vi "Simple Spectrometer Demo.vi"() -> ()   [LabVIEW 2010]
uses:
  C:/Users/User/Desktop/LabView/RgbDriverKit.dll
  RgbDriverKit.dll
panel:
  out "Device":string
  out "Measured spectrum":cluster{"Y":dbl[], "Y":dbl[]}[](graph)
  out "error out":errorcluster
  in  "error in (no error)":errorcluster
  out "Status":i32(ring) items=["Idle"=0, "WaitingForTrigger"=1, "TakingSpectrum"=2, "HasData"=3, "Error"=-3, "Busy"=-2, "NotReady"=-1]
  in  "Use sensitivity calibration":bool
  in  "Exposure time [sec]":dbl=0.1 format="%#_6f"
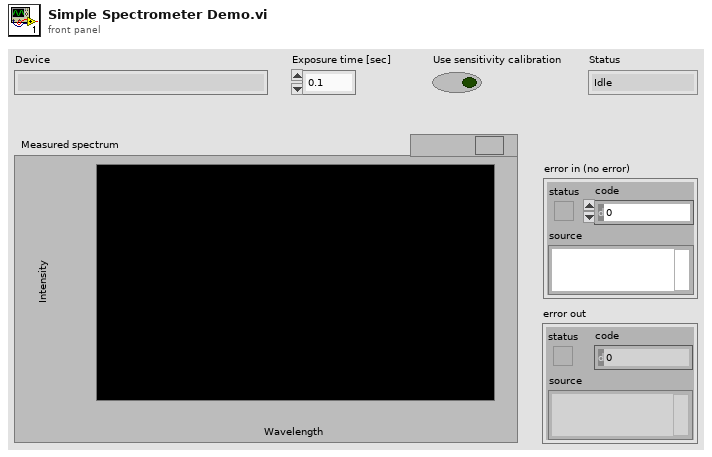
[diagram p1: front panel]
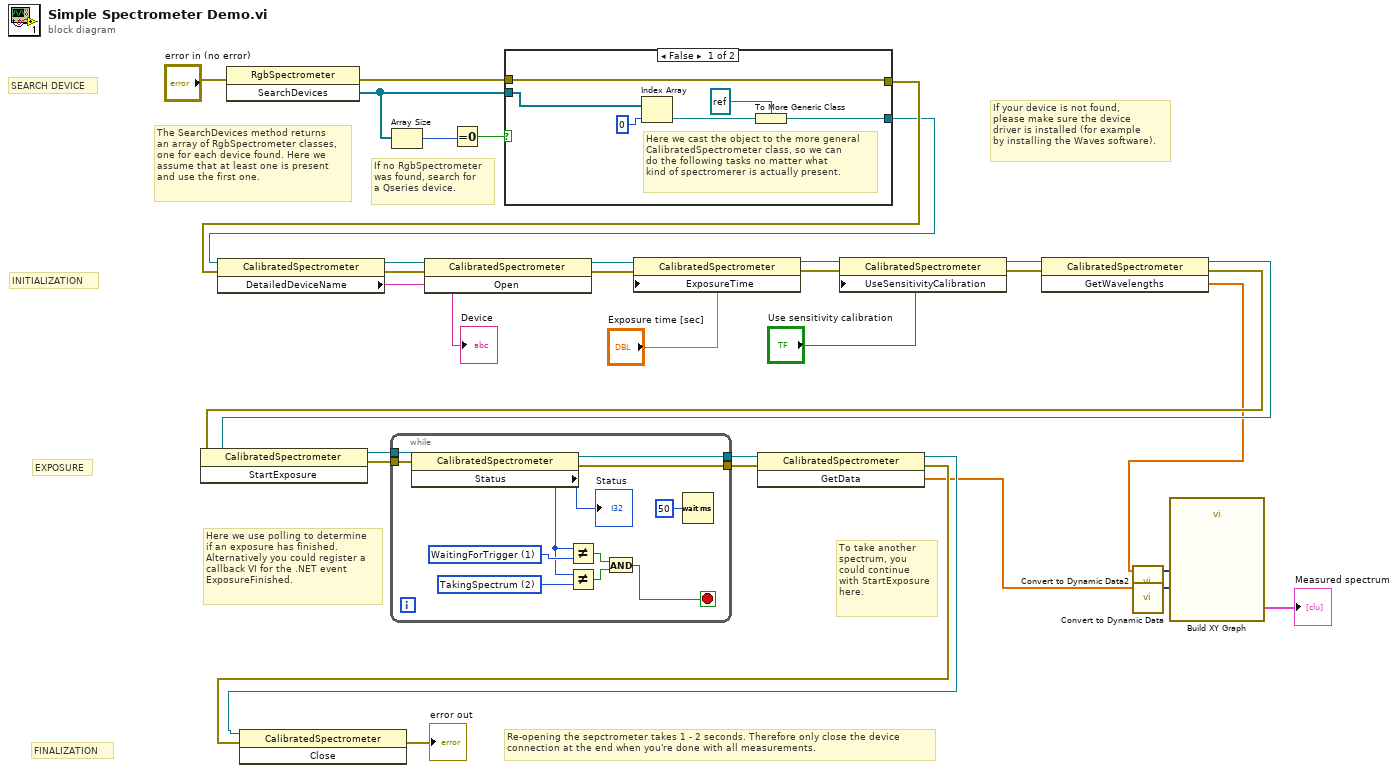
[diagram p0: block diagram]
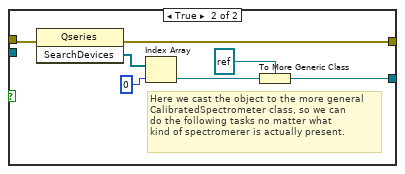
[diagram p2: hidden frame]
diagram:
  # "SEARCH DEVICE"
  # "If no RgbSpectrometer\nwas found, search for\na Qseries device."
  # "Re-opening the sepctrometer takes 1 - 2 seconds. Therefore only close the device\nconnection at the end when you're done with all measurements."
  # "To take another\nspectrum, you\ncould continue\nwith StartExposure\nhere."
  # "If your device is not found,\nplease make sure the device\ndriver is installed (for example\nby installing the Waves software)."
  # "FINALIZATION"
  # "EXPOSURE"
  # "INITIALIZATION"
  # "Here we use polling to determine\nif an exposure has finished.\nAlternatively you could register a\ncallback VI for the .NET event\nExposureFinished."
  # "The SearchDevices method returns\nan array of RgbSpectrometer classes,\none for each device found. Here we\nassume that at least one is present\nand use the first one."
  n1 = invoke class="RgbSpectrometer" method="SearchDevices"(error in="error in (no error)") -> (error out=w6:errorcluster, "SearchDevices"=w5:refnum<k24>[])  [unwired: 2 in, 1 out]
  n2 = Array Size(array=w5) -> (size(s)=w3:i32)
  n3 = Equal To 0?(x=w3) -> (x = 0?=w4:bool)
  n4 = case shown="False" w4 {
    tunnel: w6 -> [w35 w45]
    tunnel: w5 -> [w34 _]
    tunnel: [w33 w39] -> w1
    tunnel: [w35 w42] -> w2
    frame False {
      # "Here we cast the object to the more general\nCalibratedSpectrometer class, so we can\ndo the following tasks no matter what\nkind of spectromerer is actually present."
      n5 = Index Array(array=w34, index=0) -> (element=w37:refnum<k24>)
      n6 = To More Generic Class(target class=refnum<k24> refnum, reference=w37) -> (generic class reference=w33:refnum<k24>)
    }
    frame True {
      # "Here we cast the object to the more general\nCalibratedSpectrometer class, so we can\ndo the following tasks no matter what\nkind of spectromerer is actually present."
      n7 = invoke class="Qseries" method="SearchDevices"(error in=w45) -> (error out=w42:errorcluster, "SearchDevices"=w44:refnum<k24>[])  [unwired: 2 in, 1 out]
      n8 = Index Array(array=w44, index=0) -> (element=w41:refnum<k24>)
      n9 = To More Generic Class(target class=refnum<k24> refnum, reference=w41) -> (generic class reference=w39:refnum<k24>)
    }
  }
  n10 = property class="CalibratedSpectrometer"(reference=w1, error in=w2) -> (reference out=w11:refnum<k24>, error out=w10:errorcluster, "DetailedDeviceName"=→"Device":string)
  n11 = invoke class="CalibratedSpectrometer" method="Open"(reference=w11, error in=w10) -> (reference out=w31:refnum<k24>, error out=w32:errorcluster)  [unwired: 1 in, 1 out]
  n12 = property class="CalibratedSpectrometer"(reference=w31, error in=w32, "ExposureTime"="Exposure time [sec]") -> (reference out=w29:refnum<k24>, error out=w28:errorcluster)
  n13 = property class="CalibratedSpectrometer"(reference=w29, error in=w28, "UseSensitivityCalibration"="Use sensitivity calibration") -> (reference out=w16:refnum<k24>, error out=w15:errorcluster)
  n14 = invoke class="CalibratedSpectrometer" method="GetWavelengths"(reference=w16, error in=w15) -> (reference out=w13:refnum<k24>, error out=w14:errorcluster, "GetWavelengths"=w8:dbl[])  [unwired: 1 in]
  n15 = invoke class="CalibratedSpectrometer" method="StartExposure"(reference=w13, error in=w14) -> (reference out=w26:refnum<k24>, error out=w25:errorcluster)  [unwired: 1 in, 1 out]
  n16 = while {
    tunnel: w26 -> [w55]
    tunnel: w25 -> [w54]
    tunnel: [w53] -> w24
    tunnel: [w52] -> w23
    stop <- w47 stop-if-true
    w50 = 2 items=["Idle"=0, "WaitingForTrigger"=1, "TakingSpectrum"=2, "HasData"=3, "Error"=-3, "Busy"=-2, "NotReady"=-1] ("Status")
    w51 = 1 items=["Idle"=0, "WaitingForTrigger"=1, "TakingSpectrum"=2, "HasData"=3, "Error"=-3, "Busy"=-2, "NotReady"=-1] ("Status")
    n17 = property class="CalibratedSpectrometer"(reference=w55, error in=w54) -> (reference out=w53:refnum<k24>, error out=w52:errorcluster, "Status"=w46:i32)
    "Status" <- w46
    n18 = Not Equal?(x=w46, y=w51) -> (x != y?=w49:bool)
    n19 = Not Equal?(x=w46, y=w50) -> (x != y?=w48:bool)
    n20 = And(x=w49, y=w48) -> (x .and. y?=w47:bool)
    n21 = Wait (ms)(milliseconds to wait=u32 50) -> ()  [unwired: 1 out]
  }
  n22 = invoke class="CalibratedSpectrometer" method="GetData"(reference=w24, error in=w23) -> (reference out=w21:refnum<k24>, error out=w22:errorcluster, "GetData"=w7:sgl[])  [unwired: 1 in]
  n23 = invoke class="CalibratedSpectrometer" method="Close"(reference=w21, error in=w22) -> (error out=→"error out":errorcluster)  [unwired: 1 in, 2 out]
  n24 = call "Convert to Dynamic Data2"("Array"=w8) -> ("Dynamic Data Type"=w12:dynamicdata)  [unwired: 3 in]
  n25 = call "Convert to Dynamic Data"("Array"=w7) -> ("Dynamic Data Type"=w17:dynamicdata)  [unwired: 3 in]
  n26 = call "Build XY Graph"("Y Input"=w17, "X Input"=w12) -> ("XY Graph"=→"Measured spectrum":cluster{"Y":dbl[], "Y":dbl[]}[])  [unwired: 3 in, 6 out]
